vi "Drive to Image Height - Toward Key (Autonomous).vi"(1 "Execute":bool=TRUE, 2 "Image Height (Pixels)":dbl=10.0, 3 "Percent Velocity":dbl=0.8) -> (4 "Done Executing":bool)   [LabVIEW 2012]
uses:
  Globals/Autonomous Joystick Emulation.vi
  Globals/Image Height.vi
  Globals/Alignment Error.vi
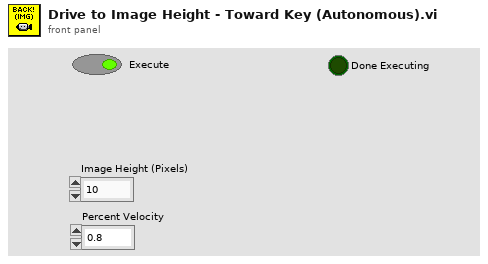
[diagram p1: front panel]
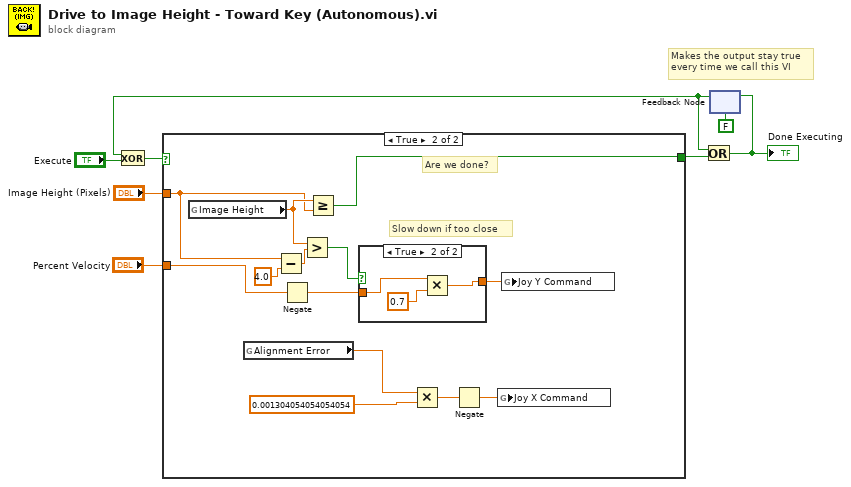
[diagram p0: block diagram]
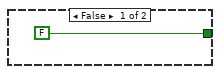
[diagram p2: hidden frame]
diagram:
  # "Makes the output stay true\nevery time we call this VI"
  n1 = feedback #1(FALSE) -> (w3:bool)
  n2 = Exclusive Or(1:"Execute", 2:w3) -> (0:w8:bool)
  n3 = case shown="True" w8 {
    tunnel: [FALSE w22] -> w6
    tunnel: "Percent Velocity" -> [_ w19]
    tunnel: "Image Height (Pixels)" -> [_ w15]
    frame False {
    }
    frame True {
      # "Slow down if too close"
      # "Are we done?"
      n4 = global read "Image Height.vi" "Image Height"() -> (w17:dbl)
      n5 = global read "Alignment Error.vi" "Alignment Error"() -> (w12:dbl)
      n6 = Subtract(x=w15, y=4.0) -> (x-y=w16:dbl)
      n7 = Negate(x=w19) -> (-x=w14:dbl)
      n8 = Greater?(x=w17, y=w16) -> (0:w21:bool)
      n9 = Greater Or Equal?(x=w17, y=w15) -> (x >= y?=w22:bool)
      n10 = case shown="True" w21 {
        tunnel: [w23 w24] -> w20
        tunnel: w14 -> [w23 w26]
        frame False {
        }
        frame True {
          n11 = Multiply(x=w26, y=0.7) -> (x*y=w24:dbl)
        }
      }
      n12 = Multiply(x=w12, y=0.001304054054054054 ("Proportional Gain (Alignment)")) -> (x*y=w11:dbl)
      n13 = Negate(x=w11) -> (-x=w10:dbl)
      n14 = global write "Autonomous Joystick Emulation.vi" "Joy X Command"(w10) -> ()
      n15 = global write "Autonomous Joystick Emulation.vi" "Joy Y Command"(w20) -> ()
    }
  }
  n16 = Or(x=w3, y=w6) -> (x .or. y?=w2:bool)
  "Done Executing" <- w2
  n17 = feedback-in #1(w2) -> ()
